vi "Read Current.vi"   [LabVIEW 2020, in "Keithley 2600 Series.lvlib"]
doc: "Performs a voltage sweep with current measured at every point."
uses:
  <instrlib>/Keithley 2600 Series/Keithley 2600 Series.lvlib
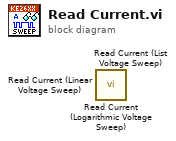
[diagram p0: block diagram]
diagram:
  n1 = call <instrlib>:"Read Current (Logarithmic Voltage Sweep).vi"() -> ()  [unwired: 9 in, 3 out]
  n2 = call <instrlib>:"Read Current (List Voltage Sweep).vi"() -> ()  [unwired: 9 in, 3 out]
  n3 = call <instrlib>:"Read Current (Linear Voltage Sweep).vi"() -> ()  [unwired: 9 in, 3 out]
